vi "Configure Limit Test.vi"(7 "Limit Test (T: Enable)":bool=TRUE, 8 "error in (no error)":errorcluster, 9 "Calculate Block (1: Calculate Block 1)":i32(ring)=1 items=["Calculate Block 1"=1, "Calculate Block 2"=2, "Calculate Block 3"=3, "Calculate Block 4"=4], 10 "FCO Auto Clear (0: OFF)":i32(ring) items=["OFF", "ON", "ONCE"], 11 "VISA resource name":refnum<visa-resource-name>) -> (0 "error out":errorcluster, 3 "VISA resource name out":refnum<visa-resource-name>)   [LabVIEW 2018, in "Agilent U2000 Series.lvlib"]
doc: "Controls when the FCO (fail counter) is cleared of any limit failures."
uses:
  Agilent U2000 Series.lvlib
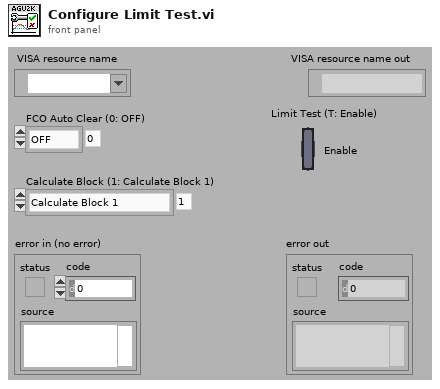
[diagram p1: front panel]
types:
  T1 = typedef "Agilent U2000 Series.lvlib/Extended User Data.ctl" = cluster{"U2000 Series Mode":u16, "Trigger Source Int/Ext":bool}
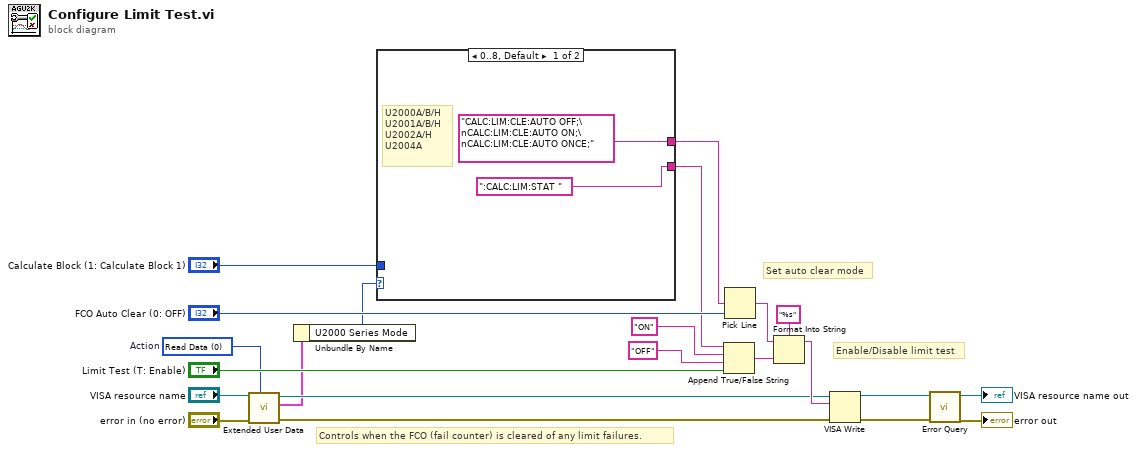
[diagram p0: block diagram]
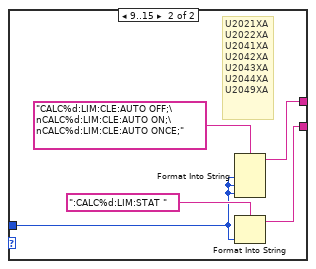
[diagram p2: hidden frame]
diagram:
  w3 = 0 items=["Read Data", "Write Data", "Clear Data", "Clear ALL Data"]  # Action
  # "Controls when the FCO (fail counter) is cleared of any limit failures."
  # "Enable/Disable limit test"
  # "Set auto clear mode"
  n1 = call "Extended User Data.vi"("Action (1: Write Data)"=w3, "error in (no error)"="error in (no error)", "VISA resource name"="VISA resource name") -> ("error out"=w4:errorcluster, "User Data Out"=w2:T1, "VISA resource name out"=w5:refnum<visa-resource-name>)  [unwired: 1 in, 5 out]
  n2 = Unbundle By Name(w2) -> ("U2000 Series Mode"=w1:u16)
  n3 = case shown="0..8, Default" w1 {
    tunnel: ["CALC:LIM:CLE:AUTO OFF;\nCALC:LIM:CLE:AUTO ON;\nCALC:LIM:CLE:AUTO ONCE;" w26] -> w10
    tunnel: [":CALC:LIM:STAT " w27] -> w9
    tunnel: "Calculate Block (1: Calculate Block 1)" -> [_ w25]
    frame 0..8, Default {
      # "U2000A/B/H\nU2001A/B/H\nU2002A/H\nU2004A"
    }
    frame 9..15 {
      # "U2021XA\nU2022XA\nU2041XA\nU2042XA\nU2043XA\nU2044XA\nU2049XA"
      n4 = Format Into String(format string="CALC%d:LIM:CLE:AUTO OFF;\nCALC%d:LIM:CLE:AUTO ON;\nCALC%d:LIM:CLE:AUTO ONCE;", w25, w25, w25) -> (resulting string=w26:string)  [unwired: 2 in, 1 out]
      n5 = Format Into String(format string=":CALC%d:LIM:STAT ", w25) -> (resulting string=w27:string)  [unwired: 2 in, 1 out]
    }
  }
  n6 = Append True/False String(1:"Limit Test (T: Enable)", 2:"OFF" ("false string"), 3:"ON" ("true string"), 4:w9) -> (0:w17:string)
  n7 = Pick Line(multi-line string=w10, line index="FCO Auto Clear (0: OFF)") -> (output string=w19:string)  [unwired: 1 out]
  n8 = Format Into String(format string="%s", initial string=w19, w17) -> (resulting string=w11:string)  [unwired: 1 in, 1 out]
  n9 = VISA Write(VISA resource name=w5, write buffer=w11, error in (no error)=w4) -> (VISA resource name out=w15:refnum<visa-resource-name>, error out=w14:errorcluster)  [unwired: 1 out]
  n10 = call "Error Query.vi"("error in (no error)"=w14, "VISA resource name"=w15) -> ("error out"=→"error out":errorcluster, "VISA resource name out"=→"VISA resource name out":refnum<visa-resource-name>)  [unwired: 8 out]
